vi "Create Front Panel Events.vi"(8 "error in (no error)":errorcluster, 11 "Viewer in":refnum<class "Viewer.lvclass">) -> (0 "error out":errorcluster, 3 "Viewer out":refnum<class "Viewer.lvclass">)   [LabVIEW 2018, in "Viewer.lvlib" / "Viewer.lvclass"]
uses:
  Viewer.lvclass
  Viewer.lvclass/Viewer.ctl
  UI Window/UI Window.lvclass
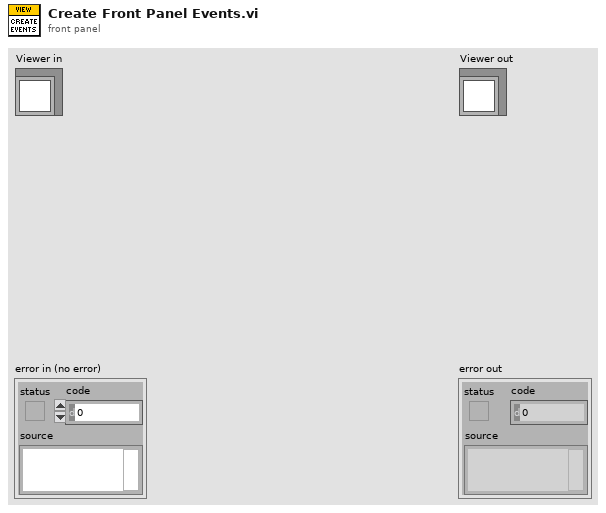
[diagram p1: front panel]
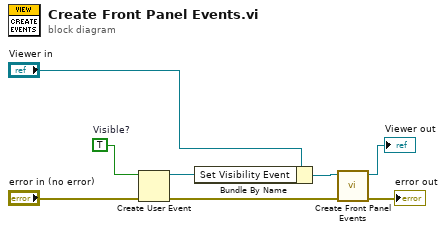
[diagram p0: block diagram]
diagram:
  w2 = TRUE  # Visible?
  n1 = Create User Event(user event datatype=w2, error in="error in (no error)") -> (user event=w3:refnum<user-event>, error out=w4:errorcluster)
  n2 = Bundle By Name(cluster="Viewer in", "Set Visibility Event"=w3) -> (w5:refnum<class "Viewer.lvclass">)
  n3 = call-parent "Create Front Panel Events.vi"("error in (no error)"=w4, "UI Window in"=w5) -> ("error out"=→"error out":errorcluster, "UI Window out"=→"Viewer out":refnum<class "Viewer.lvclass">)  [unwired: 8 in]
